vi "LinearInterpolation.vi"(0 "X":dbl, 5 "x1":dbl, 7 "y1":dbl, 9 "x2":dbl, 11 "y2":dbl) -> (8 "Value":dbl)   [LabVIEW 2016]
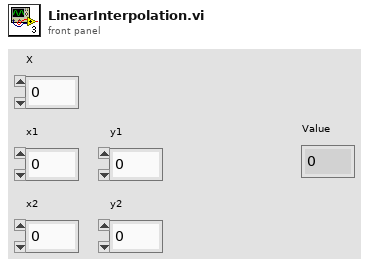
[diagram p1: front panel]
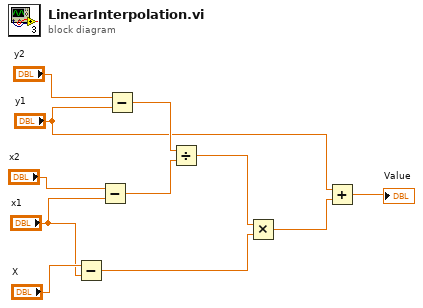
[diagram p0: block diagram]
diagram:
  n1 = Subtract(x="X", y="x1") -> (x-y=w4:dbl)
  n2 = Subtract(x="x2", y="x1") -> (x-y=w8:dbl)
  n3 = Subtract(x="y2", y="y1") -> (x-y=w9:dbl)
  n4 = Divide(x=w9, y=w8) -> (x/y=w5:dbl)
  n5 = Multiply(x=w5, y=w4) -> (x*y=w2:dbl)
  n6 = Add(x="y1", y=w2) -> (x+y=→"Value":dbl)
